vi "hwOperation_Start DAQ.vi"(7 "hwType":string, 8 "error in":errorcluster, 10 "Devs Info in":T1[](array[typedef]), 11 "hwDriverRef in":T3) -> (0 "error out":errorcluster, 2 "Devs Info out":T1[](array[typedef]), 3 "hwDriverRef out":T3)   [LabVIEW 2016]
uses:
  DAQ-Config/Controls/PSCHN_Card Para.ctl
  DAQ-Config/Controls/PSCHN_Channel Para.ctl
  QX/hw_QX_hwDriverRef.ctl
  C:/Users/CL/Desktop/ZcDAQprj0811/ZcDAQprj/Modules/DAQ-Device/Hardware Drivers/QX/HBM LabVIEW Driver/DLLs/Hbm.Api.Common.dll
  QX/HBM LabVIEW Driver/DLLs/Hbm.Api.Common.dll
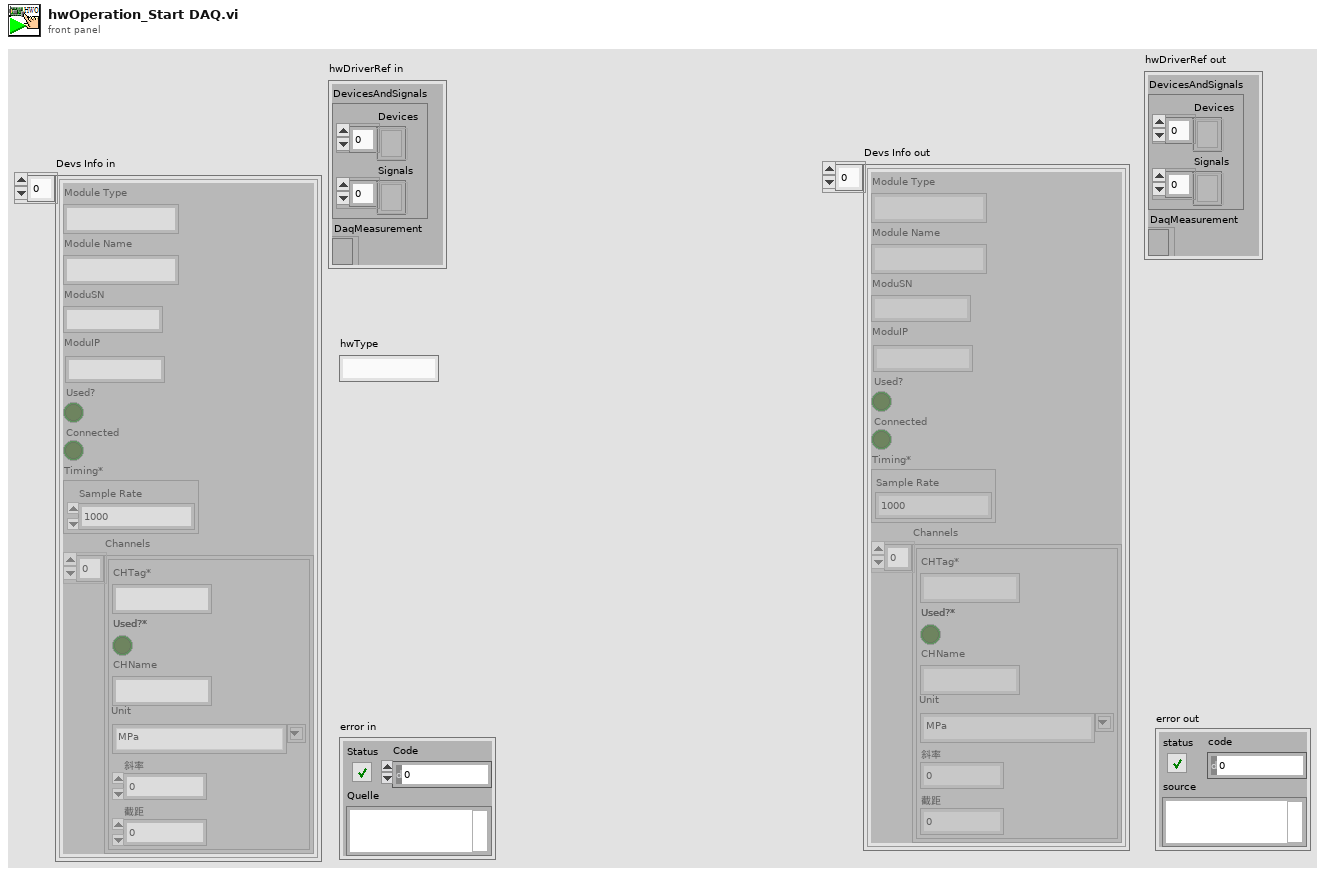
[diagram p1: front panel]
types:
  T1 = typedef "PSCHN_Card Para.ctl" = cluster{"Module Type":string, "Module Name":string, "ModuSN":string, "ModuIP":string, "Used?":bool, "Connected":bool, "Timing*":cluster{"Sample Rate":dbl}, "Channels":T2[]}
  T2 = typedef "PSCHN_Channel Para.ctl" = cluster{"CHTag*":string, "Used?*":bool, "CHName":string, "Unit":string, "斜率":dbl, "截距":dbl}
  T3 = typedef "hw_QX_hwDriverRef.ctl" = cluster{"DevicesAndSignals":cluster{"Devices":refnum<k24>[], "Signals":refnum<k24>[]}, "DaqMeasurement":refnum<k24>}
  T4 = cluster{"Devices":refnum<k24>[], "Signals":refnum<k24>[]}
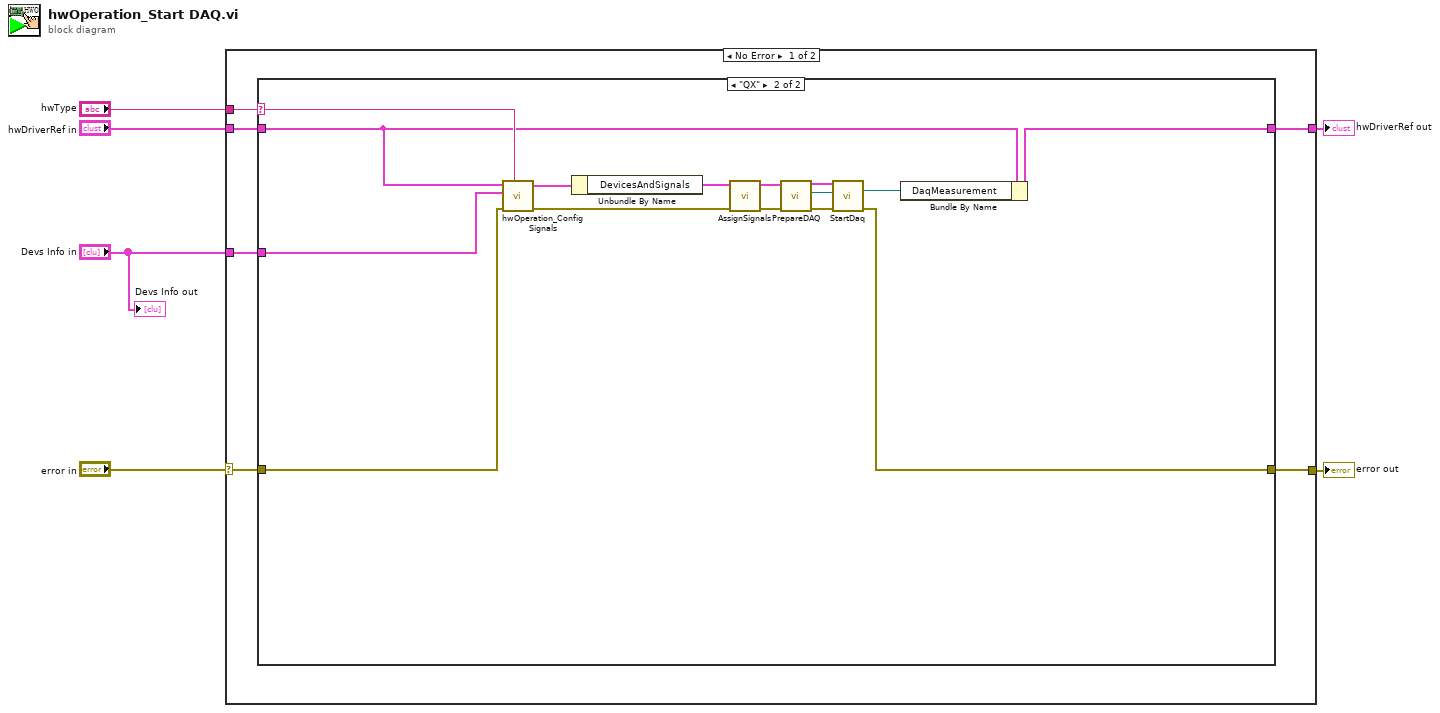
[diagram p0: block diagram]
diagram:
  n1 = case shown="No Error" "error in" {
    selector: "error in" -> [w11 w31]
    tunnel: [w12 w31] -> w5
    tunnel: "hwType" -> [w10 _]
    tunnel: "hwDriverRef in" -> [w9 w30]
    tunnel: [w8 w30] -> w2
    tunnel: "Devs Info in" -> [w7 _]
    frame No Error {
      n2 = case shown="\"QX\"" w10 {
        selector: w10 -> [_ w22]
        tunnel: [w14 w23] -> w12
        tunnel: w11 -> [w14 w24]
        tunnel: w9 -> [w13 w17]
        tunnel: [w13 w15] -> w8
        tunnel: w7 -> [_ w21]
        frame "Simulation", Default {
        }
        frame "QX" {
          n3 = call "hwOperation_Config Signals.vi"("hwType"=w22, "error in"=w24, "Devs Info in"=w21, "hwDriverRef in"=w17) -> ("error out"=w29:errorcluster, "hwDriverRef out"=w19:T3)  [unwired: 6 in]
          n4 = Unbundle By Name(w19) -> ("DevicesAndSignals"=w18:T4)
          n5 = call "AssignSignals.vi"("Error in"=w29, "DevicesAndSignals"=w18) -> ("Error out"=w25:errorcluster, "DevicesAndSignals"=w26:T4)  [unwired: 8 in]
          n6 = call "PrepareDAQ.vi"("Error in"=w25, "DevicesAndSignals"=w26) -> ("Error out"=w27:errorcluster, "DaqMeasurement"=w20:refnum<k24>, "DevicesAndSignals"=w28:T4)  [unwired: 7 in]
          n7 = call "StartDaq.vi"("DevicesAndSignals"=w28, "DaqMeasurement"=w20, "Error in"=w27) -> ("DaqMeasurement"=w16:refnum<k24>, "Error out"=w23:errorcluster)  [unwired: 9 in, 2 out]
          n8 = Bundle By Name(cluster=w17, "DaqMeasurement"=w16) -> (w15:T3)
        }
      }
    }
    frame Error {
    }
  }
  "error out" <- w5
  "hwDriverRef out" <- w2
  "Devs Info out" <- "Devs Info in"
